vi "VI Tree.vi"   [LabVIEW 2012, in "Phidget Encoder.lvlib"]
doc: "${Encoder:VITreeHeader}"
uses:
  <instrlib>/Phidgets/Phidget Encoder/Phidget Encoder.lvlib
  <instrlib>/Phidgets/Phidget Encoder/Public/EncoderStart.vi
  <instrlib>/Phidgets/Phidget Encoder/Public/EncoderOpen.vi
  <instrlib>/Phidgets/Phidget Encoder/Public/EncoderClose.vi
panel:
  # "(c) 2015 Phidgets Inc..  ALL RIGHTS RESERVED."
  # "SEE DIAGRAM\nFOR VI TREE."
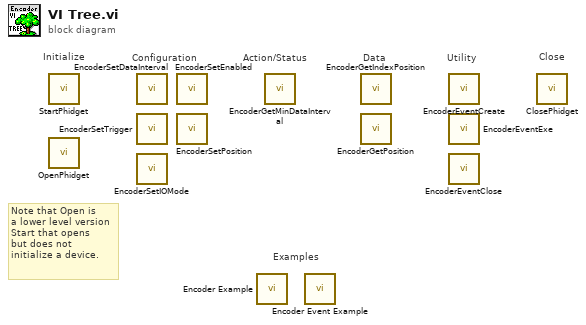
[diagram p0: block diagram]
diagram:
  # "Note that Open is\na lower level version\nStart that opens\nbut does not \ninitialize a device."
  # "Examples"
  # "Configuration"
  # "Utility"
  # "Data"
  # "Action/Status"
  # "Close"
  # "Initialize"
  n1 = call-poly <instrlib>:"StartPhidget.vi"() -> ()  [unwired: 12 in, 4 out]
  n2 = call-poly <instrlib>:"OpenPhidget.vi"() -> ()  [unwired: 8 in, 4 out]
  n3 = call <instrlib>:"EncoderSetDataInterval.vi"() -> ()  [unwired: 9 in, 2 out]
  n4 = call <instrlib>:"EncoderSetTrigger.vi"() -> ()  [unwired: 9 in, 2 out]
  n5 = call <instrlib>:"EncoderSetIOMode.vi"() -> ()  [unwired: 9 in, 2 out]
  n6 = call <instrlib>:"EncoderSetEnabled.vi"() -> ()  [unwired: 9 in, 2 out]
  n7 = call <instrlib>:"EncoderSetPosition.vi"() -> ()  [unwired: 9 in, 2 out]
  n8 = call <instrlib>:"Encoder Example.vi"() -> ()  [unwired: 12 in]
  n9 = call <instrlib>:"EncoderGetMinDataInterval.vi"() -> ()  [unwired: 8 in, 3 out]
  n10 = call <instrlib>:"Encoder Event Example.vi"() -> ()  [unwired: 12 in]
  n11 = call <instrlib>:"EncoderGetIndexPosition.vi"() -> ()  [unwired: 8 in, 3 out]
  n12 = call <instrlib>:"EncoderGetPosition.vi"() -> ()  [unwired: 8 in, 3 out]
  n13 = call <instrlib>:"EncoderEventCreate.vi"() -> ()  [unwired: 9 in, 3 out]
  n14 = call <instrlib>:"EncoderEventExe.vi"() -> ()  [unwired: 11 in, 9 out]
  n15 = call <instrlib>:"EncoderEventClose.vi"() -> ()  [unwired: 10 in, 2 out]
  n16 = call-poly <instrlib>:"ClosePhidget.vi"() -> ()  [unwired: 11 in, 1 out]
